vi "set value for key.vi"(8 "error in":errorcluster, 9 "value":string, 10 "key":string, 11 "fixed channel configuration in":refnum<class "fixed channel configuration.lvclass">) -> (0 "error out":errorcluster, 3 "fixed channel configuration out":refnum<class "fixed channel configuration.lvclass">)   [LabVIEW 2013, in "fixed channel configuration.lvclass"]
uses:
  fixed channel configuration.lvclass
  fixed channel configuration.lvclass/fixed channel configuration.ctl
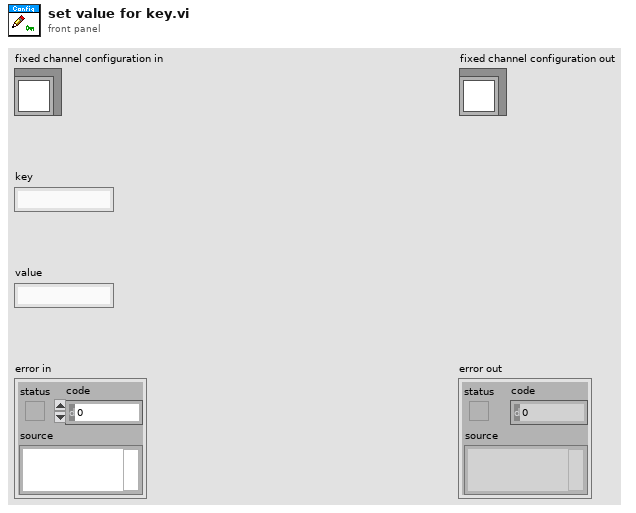
[diagram p1: front panel]
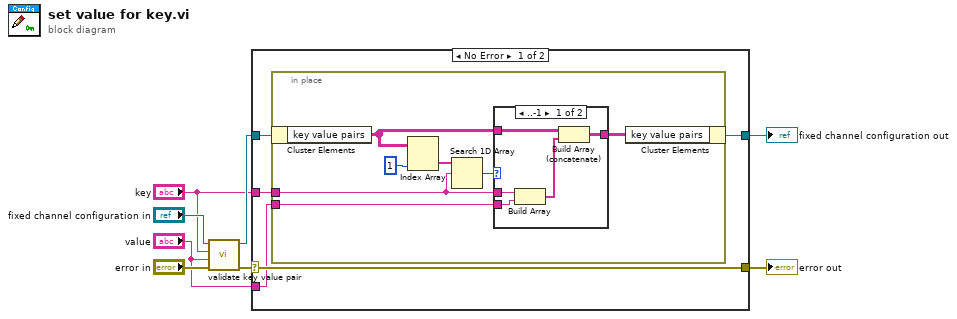
[diagram p0: block diagram]
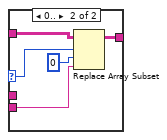
[diagram p2: hidden frame]
diagram:
  n1 = call-dynamic "validate key value pair.vi"("error in"="error in", "value"="value", "key"="key", "fixed channel configuration in"="fixed channel configuration in") -> ("error out"=w6:errorcluster, "fixed channel configuration out"=w4:refnum<class "fixed channel configuration.lvclass">)  [unwired: 6 in]
  n2 = case shown="No Error" w6 {
    selector: w6 -> [w13 w32]
    tunnel: [w13 w32] -> w5
    tunnel: [w11 w31] -> w3
    tunnel: w4 -> [w12 w31]
    tunnel: "key" -> [w10 _]
    tunnel: "value" -> [w9 _]
    frame No Error {
      n3 = in-place {
        in-place-border: w10 -> [w15]
        in-place-border: w9 -> [w16]
        n4 = in-place-cluster #1(w12) -> ("key value pairs"=w14:string[][])
        n5 = Index Array(array=w14, index (col)=1 ("disabled index (col)")) -> (element=w19:string[])  [unwired: 1 in]
        n6 = Search 1D Array(1D array=w19, element=w15) -> (index of element=w18:i32)  [unwired: 1 in]
        n7 = case shown="..-1" w18 {
          selector: w18 -> [_ w27]
          tunnel: w14 -> [w25 w30]
          tunnel: [w24 w29] -> w17
          tunnel: w16 -> [w22 w26]
          tunnel: w15 -> [w23 _]
          frame ..-1 {
            n8 = Build Array(w23, w22) -> (w21:string[])
            n9 = Build Array (concatenate)(w25, w21) -> (w24:string[][])
          }
          frame 0.. {
            n10 = Replace Array Subset(array=w30, new element=w26, index (row)=w27, index (col)=0 ("disabled index (col)")) -> (w29:string[][])
          }
        }
        n11 = in-place-cluster #1("key value pairs"=w17) -> (w11:refnum<class "fixed channel configuration.lvclass">)
      }
    }
    frame Error {
    }
  }
  "error out" <- w5
  "fixed channel configuration out" <- w3
